vi "Complex Inverse Matrix (LU).vi"(3 "A":T1) -> (0 "error":i32, 1 "Inverse Matrix":T1)   [LabVIEW 2017, in "NI_AALBase.lvlib"]
doc: "Finds the <B>Inverse Matrix</B>, if it exists, of the <B>Input Matrix</B>, using LU factorization."
uses:
  <vilib>/Analysis/NI_AALBase.lvlib
  <vilib>/Analysis/Matrix/Datatypes/ComplexMatrix.ctl
  <resource>/lvanlys.dll
  <vilib>/Analysis/Matrix/NI_Matrix.lvlib
panel:
  # "Complex Inverse Matrix (LU)"
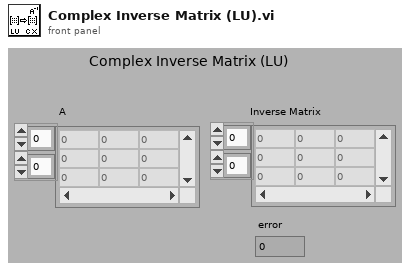
[diagram p1: front panel]
types:
  T1 = typedef "NI_Matrix.lvlib/ComplexMatrix.ctl" = cdb[][]
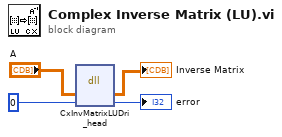
[diagram p0: block diagram]
diagram:
  n1 = dll-call lib="e:/builds/penguin/labview/branches/2017/dev/dist/resource/lvanlys.*" fn="CxInvMatrixLUDri_head"("A"="A", 0) -> ("A"=→"Inverse Matrix":T1, →"error":i32)  [unwired: 4 in, 2 out]
